vi "Get SMO HELP.vi"(8 "error in (no error)":errorcluster, 10 "Command":string, 11 "Instrument.Cryostat in":refnum<class "Instrument.Cryostat.lvclass">) -> (0 "error out":errorcluster, 2 "help cluster":T1, 3 "Instrument.Cryostat out":refnum<class "Instrument.Cryostat.lvclass">)   [LabVIEW 2019, in "Instrument.Cryostat.lvclass"]
uses:
  Instrument.Cryostat.lvclass
  <userlib>/LevyLab/Instrument Framework/subsystems/Help/typedefs/Help--cluster.ctl
  Typedefs/Cryostat.commands--enum.ctl
  Typedefs/Magnet Axis--Enum.ctl
  Typedefs/getMagnet--cluster.ctl
  Typedefs/getMagnetVector--cluster.ctl
  Typedefs/setMagnet--cluster.ctl
  Typedefs/Magnet Mode--Enum.ctl
  Typedefs/setMagnetVector--cluster.ctl
  Typedefs/getAngle--cluster.ctl
  Typedefs/setAngle--cluster.ctl
  Typedefs/getTemperature--cluster.ctl
  Typedefs/setTemperature--cluster.ctl
  Typedefs/getHeater--cluster.ctl
  Typedefs/setHeater--cluster.ctl
  Typedefs/getPressure--cluster.ctl
  <userlib>/LevyLab/Instrument Framework/Instrument/Instrument.lvclass
  <userlib>/LevyLab/Instrument Framework/subsystems/Help/Help.lvclass
  <userlib>/LevyLab/Instrument Framework/Instrument/Typedefs/Instrument.Commands--Enum.ctl
  <userlib>/LevyLab/Instrument Framework/Instrument/Typedefs/Instrument.IDN--cluster.ctl
  <vilib>/PRIrvin/JSON-Schema/JSON-Schema.lvlib
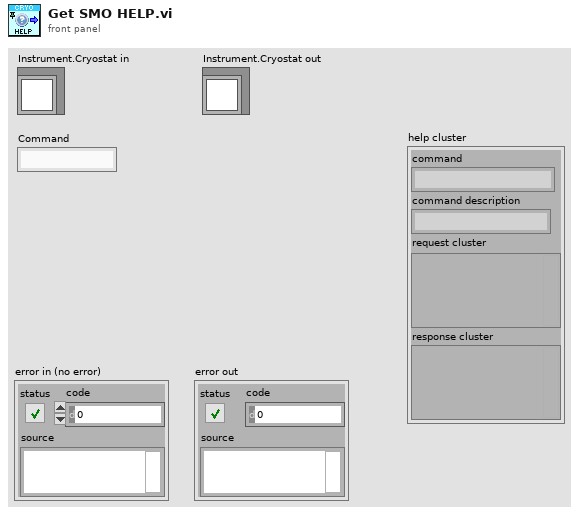
[diagram p1: front panel]
types:
  T1 = typedef "Instrument.lvlib/Help.lvclass/Help--cluster.ctl" = cluster{"command":string, "command description":string, "request cluster":variant, "response cluster":variant}
  T2 = typedef "Instrument.Cryostat.lvclass/Cryostat.commands--enum.ctl" = enum16{"getLN2Level", "getLHeLevel", "getMagnet", "getMagnetVector", "getMagnetTarget", "getMagnetVectorTarget", "setMagnet", "setMagnetVector", "getAngle", "setAngle", "getTemperature", "getTemperatureTarget", "setTemperature", "getHeater", "setHeater", "getChamber", "setChamber", "getPressure"}
  T3 = typedef "Instrument.Cryostat.lvclass/getMagnet--cluster.ctl" = cluster{"field":dbl, "status":string, "finished":bool}
  T4 = typedef "Instrument.Cryostat.lvclass/Magnet Axis--Enum.ctl" = enum16{"X", "Y", "Z"}
  T5 = typedef "Instrument.Cryostat.lvclass/getMagnetVector--cluster.ctl" = cluster{"field":dbl[], "status":string, "finished":bool}
  T6 = typedef "Instrument.Cryostat.lvclass/setMagnet--cluster.ctl" = cluster{"field":dbl, "rate":dbl, "axis":T4, "mode":T7}
  T7 = typedef "Instrument.Cryostat.lvclass/Magnet Mode--Enum.ctl" = enum16{"Persistent", "Driven"}
  T8 = typedef "Instrument.Cryostat.lvclass/setMagnetVector--cluster.ctl" = cluster{"field":dbl[], "rate":dbl}
  T9 = typedef "Instrument.Cryostat.lvclass/getAngle--cluster.ctl" = cluster{"angle":dbl, "status":string, "finished":bool}
  T10 = typedef "Instrument.Cryostat.lvclass/setAngle--cluster.ctl" = cluster{"angle":dbl, "rate":dbl, "channel":i32}
  T11 = typedef "Instrument.Cryostat.lvclass/getTemperature--cluster.ctl" = cluster{"temperature":dbl, "status":string, "finished":bool}
  T12 = typedef "Instrument.Cryostat.lvclass/setTemperature--cluster.ctl" = cluster{"temperature":dbl, "rate":dbl, "channel":i32}
  T13 = typedef "Instrument.Cryostat.lvclass/getHeater--cluster.ctl" = cluster{"current":dbl, "status":string}
  T14 = typedef "Instrument.Cryostat.lvclass/setHeater--cluster.ctl" = cluster{"current":dbl, "channel":i32}
  T15 = typedef "Instrument.Cryostat.lvclass/getPressure--cluster.ctl" = cluster{"pressure":dbl, "status":string}
  T16 = typedef "Instrument.lvlib/Instrument.lvclass/Instrument.Commands--Enum.ctl" = enum16{"ACK", "HELP", "IDN", "getAll", "getAllData"}
  T17 = typedef "Instrument.lvlib/Instrument.lvclass/Instrument.IDN--cluster.ctl" = cluster{"vendor":string, "model":string, "serial":string, "firmware":string}
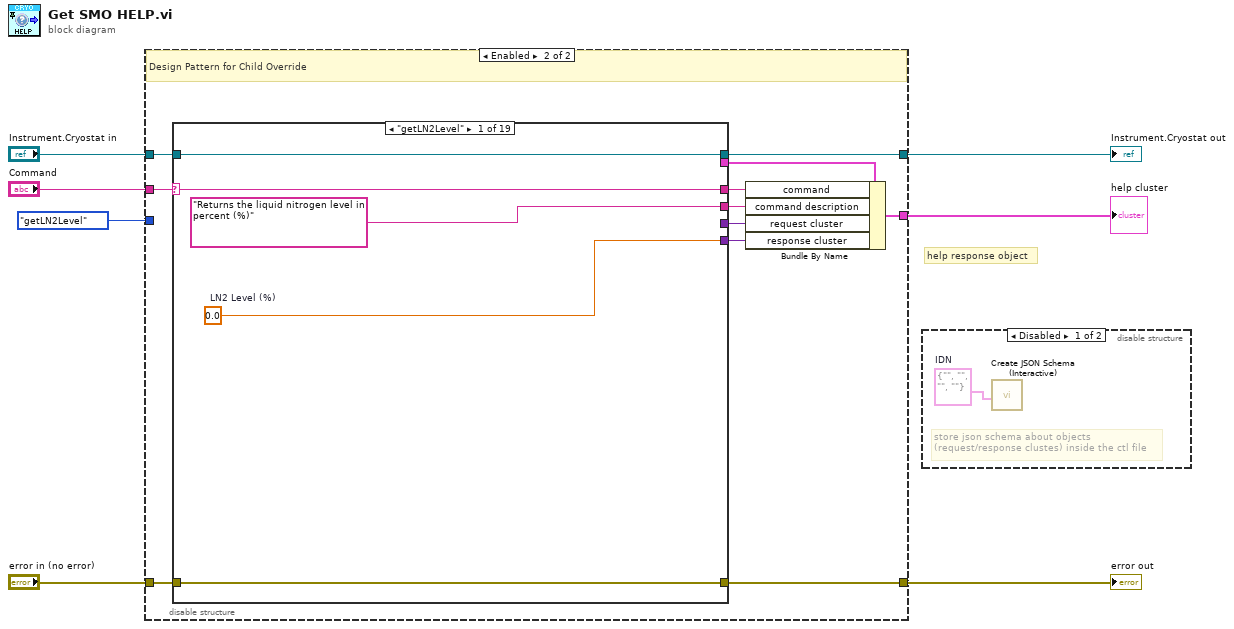
[diagram p0: block diagram]
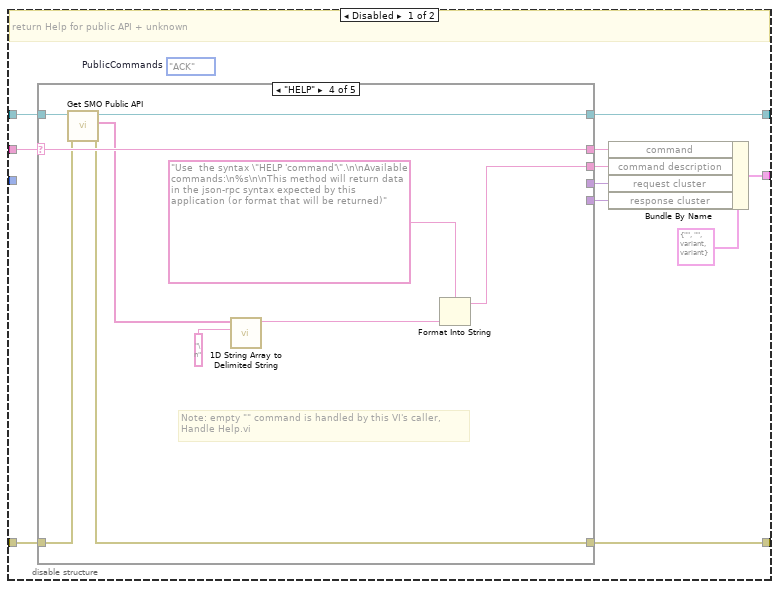
[diagram p3: hidden frame]
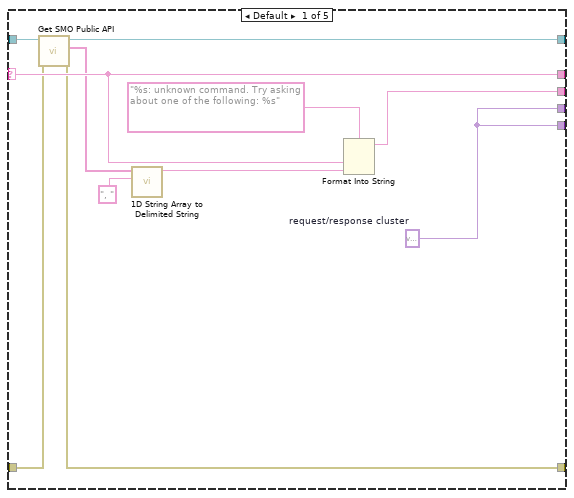
[diagram p4: hidden frame]
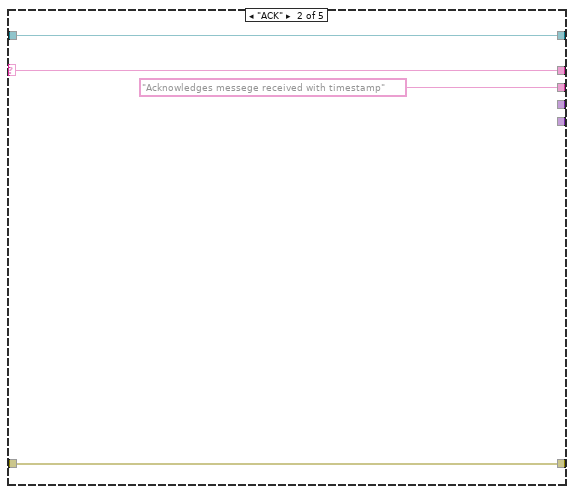
[diagram p5: hidden frame]
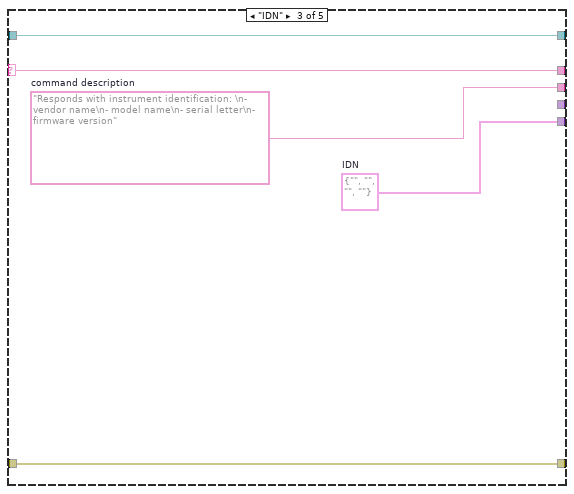
[diagram p6: hidden frame]
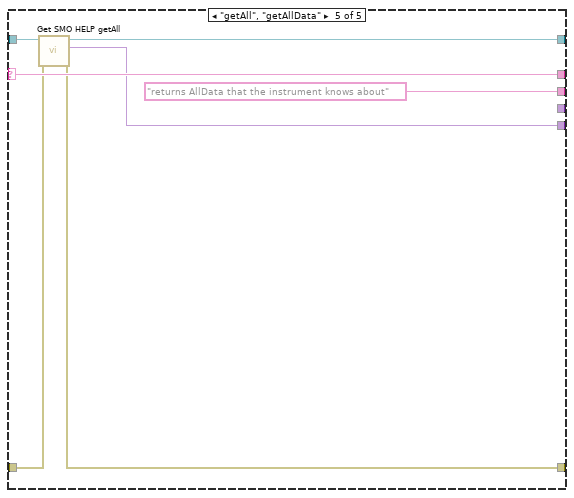
[diagram p7: hidden frame]
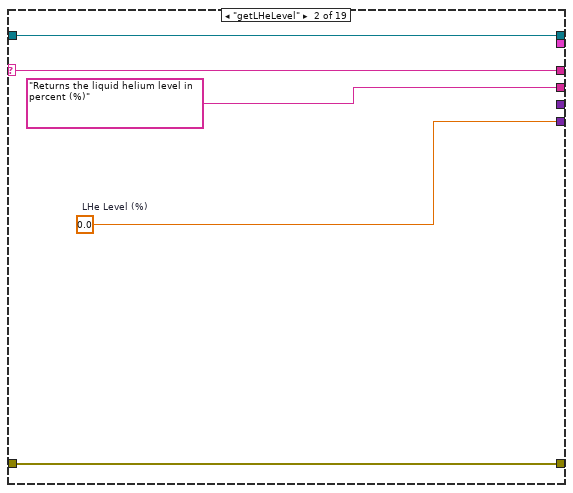
[diagram p8: hidden frame]
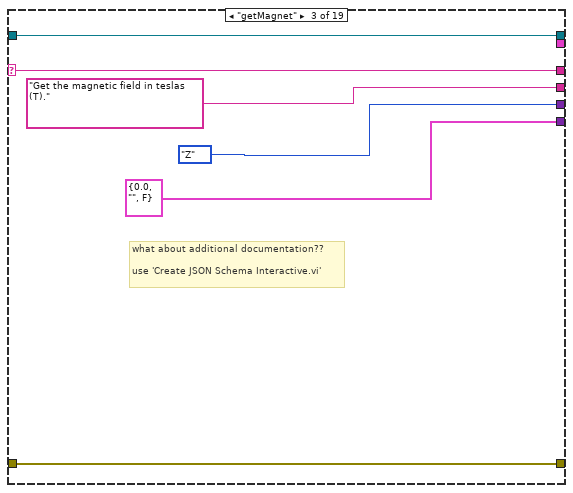
[diagram p9: hidden frame]
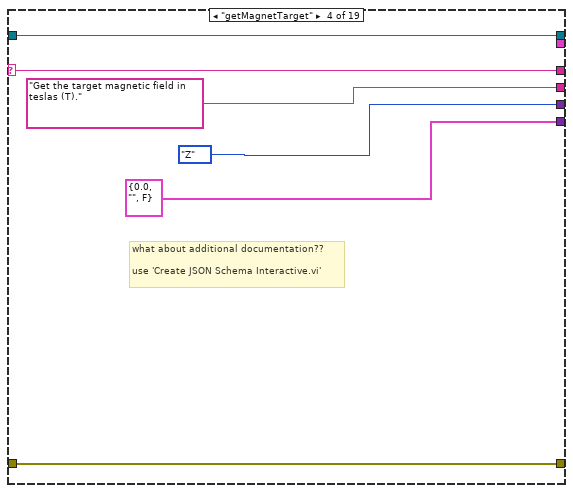
[diagram p10: hidden frame]
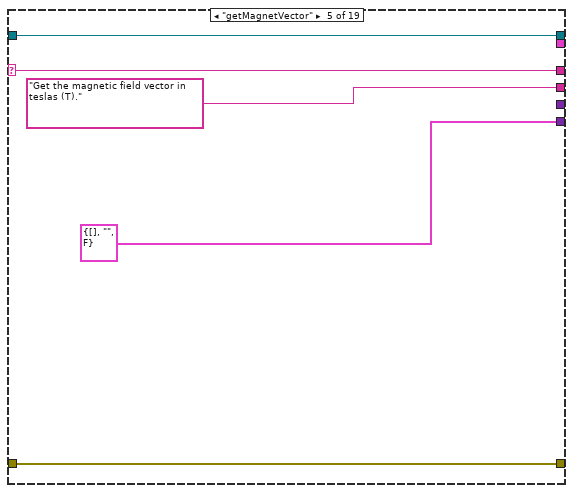
[diagram p11: hidden frame]
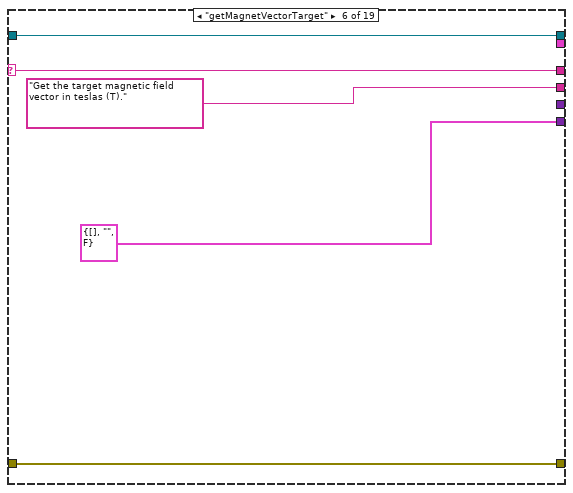
[diagram p12: hidden frame]
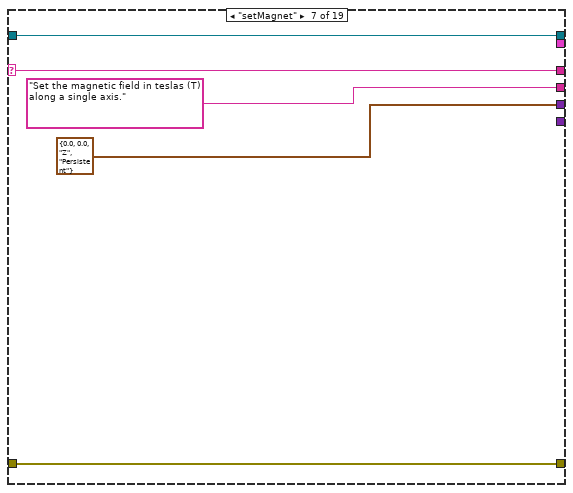
[diagram p13: hidden frame]
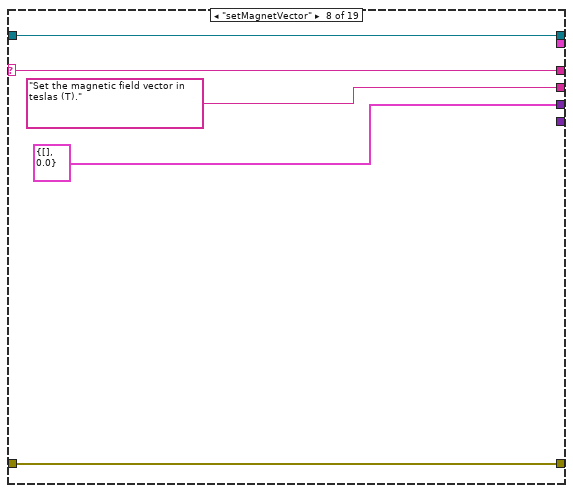
[diagram p14: hidden frame]
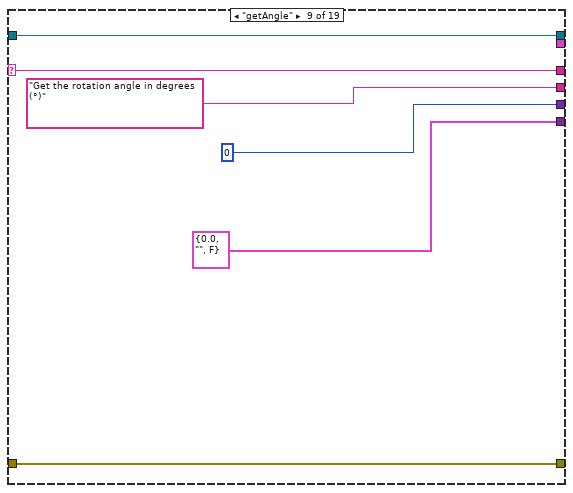
[diagram p15: hidden frame]
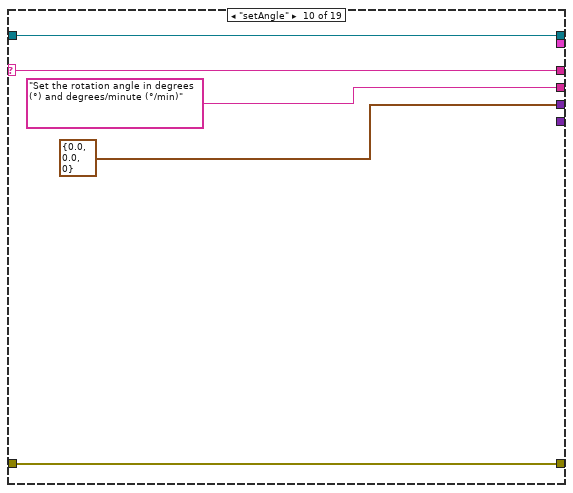
[diagram p16: hidden frame]
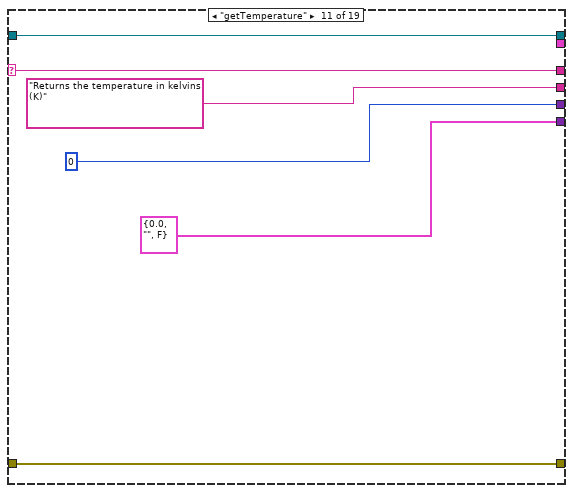
[diagram p17: hidden frame]
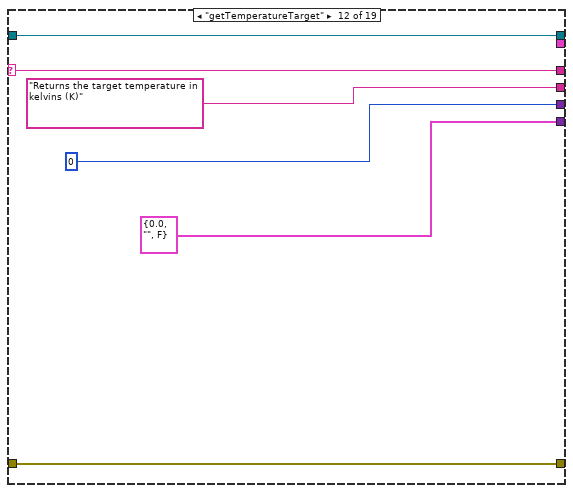
[diagram p18: hidden frame]
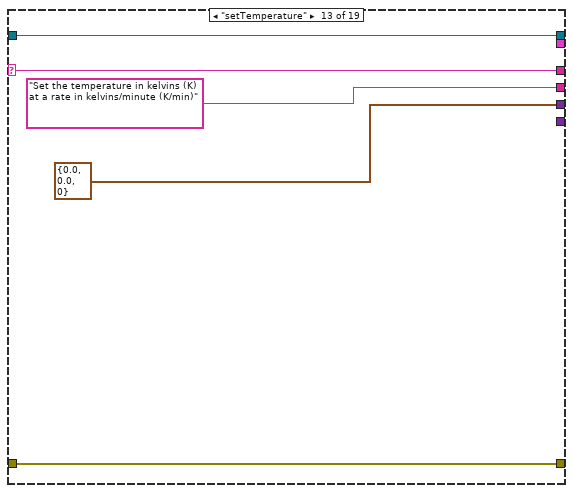
[diagram p19: hidden frame]
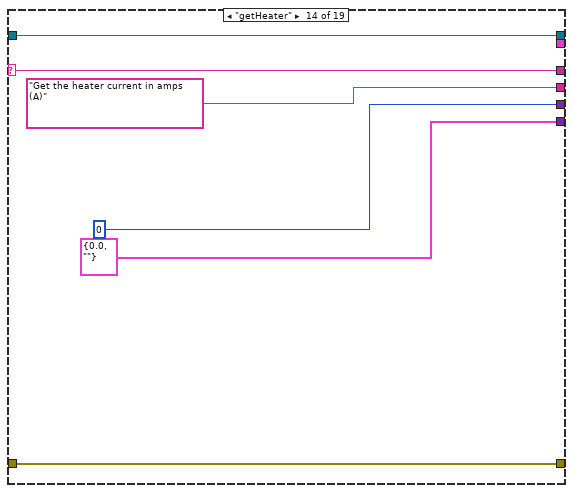
[diagram p20: hidden frame]
diagram:
  # "help response object"
  n1 = disable-structure shown="Enabled" {
    disable-tunnel: [w18 w58] -> w5
    disable-tunnel: "Instrument.Cryostat in" -> [w17 w59]
    disable-tunnel: "error in (no error)" -> [w16 w64]
    disable-tunnel: [w12 w66] -> w7
    disable-tunnel: [w9 w65] -> w6
    disable-tunnel: "Command" -> [w8 w56]
    disable-tunnel: Cryostat.commands--enum."getLN2Level" ("commands") -> [_ _]
    frame Disabled {
      (unwired) Instrument.Commands--Enum."ACK"  # PublicCommands
      # "return Help for public API + unknown"
      n2 = case shown="\"HELP\"" w8 {
        selector: w8 -> [w25 w31 w37 w45 w54]
        tunnel: w16 -> [w22 w33 w35 w42 w53]
        tunnel: [w23 w33 w35 w43 w52] -> w12
        tunnel: [w27 "Acknowledges messege received with timestamp" w38 w39 "returns AllData that the instrument knows about"] -> w14
        tunnel: [w20 _ _ _ _] -> w13
        tunnel: [w20 _ w34 _ w49] -> w11
        tunnel: [w25 w31 w37 w45 w54] -> w15
        tunnel: w17 -> [w24 w30 w36 w44 w50]
        tunnel: [w21 w30 w36 w41 w51] -> w18
        frame Default {
          w20 = variant  # request/response cluster
          n3 = call-dynamic "Get SMO Public API.vi"("error in (no error)"=w22, "Instrument.Cryostat in"=w24) -> ("error out"=w23:errorcluster, "commands"=w19:string[], "Instrument.Cryostat out"=w21:refnum<class "Instrument.Cryostat.lvclass">)  [unwired: 7 in]
          n4 = call <vilib>:"1D String Array to Delimited String.vi"("delimiter"=", ", "string array"=w19) -> ("delimited string"=w28:string)  [unwired: 9 in]
          n5 = Format Into String(format string="%s: unknown command. Try asking about one of the following: %s", w25, w28) -> (resulting string=w27:string)  [unwired: 2 in, 1 out]
        }
        frame "ACK" {
        }
        frame "IDN" {
          w34 = T17 {"vendor"="", "model"="", "serial"="", "firmware"=""}  # IDN
          w38 = "Responds with instrument identification: \n- vendor name\n- model name\n- serial letter\n- firmware version"  # command description
        }
        frame "HELP" {
          # "Note: empty \"\" command is handled by this VI's caller,\nHandle Help.vi"
          n6 = call-dynamic "Get SMO Public API.vi"("error in (no error)"=w42, "Instrument.Cryostat in"=w44) -> ("error out"=w43:errorcluster, "commands"=w40:string[], "Instrument.Cryostat out"=w41:refnum<class "Instrument.Cryostat.lvclass">)  [unwired: 7 in]
          n7 = call <vilib>:"1D String Array to Delimited String.vi"("delimiter"="\n", "string array"=w40) -> ("delimited string"=w48:string)  [unwired: 9 in]
          n8 = Format Into String(format string="Use  the syntax \"HELP 'command'\".\n\nAvailable commands:\n%s\n\nThis method will return data in the json-rpc syntax expected by this application (or format that will be returned)", w48) -> (resulting string=w39:string)  [unwired: 2 in, 1 out]
        }
        frame "getAll", "getAllData" {
          n9 = call-dynamic "Get SMO HELP getAll.vi"("error in (no error)"=w53, "Instrument in"=w50) -> ("error out"=w52:errorcluster, "getAll response cluster"=w49:variant, "Instrument out"=w51:refnum<class "Instrument.Cryostat.lvclass">)  [unwired: 7 in]
        }
      }
      n10 = Bundle By Name(cluster=T1 {"command"="", "command description"="", "request cluster"=variant, "response cluster"=variant} ("Help"), "command"=w15, "command description"=w14, "request cluster"=w13, "response cluster"=w11) -> (w9:T1)
    }
    frame Enabled {
      # "Design Pattern for Child Override"
      n11 = case shown="\"getLN2Level\"" w56 {
        selector: w56 -> [w71 w76 w82 w88 w93 w98 w103 w108 w114 w119 w125 w131 w136 w142 w147 w152 w157 w163 w172]
        tunnel: [w71 w76 w82 w88 w93 w98 w103 w108 w114 w119 w125 w131 w136 w142 w147 w152 w157 w163 w167] -> w63
        tunnel: w64 -> [w70 w75 w81 w87 w92 w97 w102 w107 w113 w118 w124 w130 w135 w141 w146 w151 w156 w162 w165]
        tunnel: [w70 w75 w81 w87 w92 w97 w102 w107 w113 w118 w124 w130 w135 w141 w146 w151 w156 w162 w164] -> w66
        tunnel: ["Returns the liquid nitrogen level in percent (%)" "Returns the liquid helium level in percent (%)" "Get the magnetic field in teslas (T)." "Get the target magnetic field in teslas (T)." "Get the magnetic field vector in teslas (T)." "Get the target magnetic field vector in teslas (T)." "Set the magnetic field in teslas (T) along a single axis." "Set the magnetic field vector in teslas (T)." "Get the rotation angle in degrees (°)" "Set the rotation angle in degrees (°) and degrees/minute (°/min)" "Returns the temperature in kelvins (K)" "Returns the target temperature in kelvins (K)" "Set the temperature in kelvins (K) at a rate in kelvins/minute (K/min)" "Get the heater current in amps (A)" "Set the heater current in amps (A)" "Returns the chamber staus" "Configure the chamber state" "Returns the chamber pressure in millibars (mbar) and pressure status." w168] -> w62
        tunnel: [_ _ Magnet_Axis--Enum."Z" ("Axis") Magnet_Axis--Enum."Z" ("Axis") _ _ T6 {"field"=0.0, "rate"=0.0, "axis"=enum."Z", "mode"=enum."Persistent"} ("Set Magnet Field") T8 {"field"=[], "rate"=0.0} ("setMagnet") 0 ("Channel") T10 {"angle"=0.0, "rate"=0.0, "channel"=0} ("Set Angle") 0 ("Channel") 0 ("Channel") T12 {"temperature"=0.0, "rate"=0.0, "channel"=0} ("Set Temperature") 0 ("Channel") T14 {"current"=0.0, "channel"=0} ("Set Temperature") _ "" ("Action") 0 ("Channel") w169] -> w61
        tunnel: [w67 w72 T3 {"field"=0.0, "status"="", "finished"=FALSE} ("getMagnet") T3 {"field"=0.0, "status"="", "finished"=FALSE} ("getMagnet") T5 {"field"=[], "status"="", "finished"=FALSE} ("getMagnet") T5 {"field"=[], "status"="", "finished"=FALSE} ("getMagnet") _ _ T9 {"angle"=0.0, "status"="", "finished"=FALSE} ("getAngle") _ T11 {"temperature"=0.0, "status"="", "finished"=FALSE} ("getTemperature") T11 {"temperature"=0.0, "status"="", "finished"=FALSE} ("getTemperature") _ T13 {"current"=0.0, "status"=""} ("getHeat") _ "" _ T15 {"pressure"=0.0, "status"=""} ("getPressure") w170] -> w60
        tunnel: w59 -> [w68 w73 w79 w85 w90 w95 w100 w105 w111 w116 w122 w128 w133 w139 w144 w149 w154 w160 w173]
        tunnel: [w68 w73 w79 w85 w90 w95 w100 w105 w111 w116 w122 w128 w133 w139 w144 w149 w154 w160 w171] -> w58
        tunnel: [_ _ _ _ _ _ _ _ _ _ _ _ _ _ _ _ _ _ w166] -> w57
        frame "getLN2Level" {
          w67 = 0.0  # LN2 Level (%)
        }
        frame "getLHeLevel" {
          w72 = 0.0  # LHe Level (%)
        }
        frame "getMagnet" {
          # "what about additional documentation??\n\nuse 'Create JSON Schema Interactive.vi'"
        }
        frame "getMagnetTarget" {
          # "what about additional documentation??\n\nuse 'Create JSON Schema Interactive.vi'"
        }
        frame "getMagnetVector" {
        }
        frame "getMagnetVectorTarget" {
        }
        frame "setMagnet" {
        }
        frame "setMagnetVector" {
        }
        frame "getAngle" {
        }
        frame "setAngle" {
        }
        frame "getTemperature" {
        }
        frame "getTemperatureTarget" {
        }
        frame "setTemperature" {
        }
        frame "getHeater" {
        }
        frame "setHeater" {
        }
        frame "getChamber" {
        }
        frame "setChamber" {
        }
        frame "getPressure" {
        }
        frame Default {
          # "need string case selector because we want to support a command not inside the enum"
          # "Replace this Get GMO HELP.vi node with \"Call Parent Method\"\nwhen using this design pattern in override"
          n12 = call-parent "Get SMO HELP.vi"("error in (no error)"=w165, "Command"=w172, "Instrument in"=w173) -> ("error out"=w164:errorcluster, "help cluster"=w166:T1, "Instrument out"=w171:refnum<class "Instrument.Cryostat.lvclass">)  [unwired: 6 in]
          n13 = Unbundle By Name(w166) -> ("command"=w167:string, "command description"=w168:string, "request cluster"=w169:variant, "response cluster"=w170:variant)
        }
      }
      n14 = Bundle By Name(cluster=w57, "command"=w63, "command description"=w62, "request cluster"=w61, "response cluster"=w60) -> (w65:T1)
    }
  }
  "Instrument.Cryostat out" <- w5
  "help cluster" <- w6
  "error out" <- w7
  n15 = disable-structure shown="Disabled" {
    frame Disabled {
      w174 = T17 {"vendor"="", "model"="", "serial"="", "firmware"=""}  # IDN
      # "store json schema about objects\n(request/response clustes) inside the ctl file"
      n16 = call <vilib>:"Create JSON Schema (Interactive).vi"("LV Object"=w174) -> ()  [unwired: 9 in, 2 out]
    }
    frame Enabled {
    }
  }
